vi "Insert UI into Subpanel.vi"(8 "error in":errorcluster, 11 "Philips Subpanel in":refnum<class "Flex UI Subpanel.lvclass">) -> (0 "error out":errorcluster, 3 "Philips Subpanel out":refnum<class "Flex UI Subpanel.lvclass">)   [LabVIEW 2014, in "Flex UI Subpanel.lvclass"]
uses:
  Flex UI Subpanel.lvclass
  Flex UI Subpanel.lvclass/Flex UI Subpanel.ctl
  Flex UI (Parent)/Flex UI.lvclass/Flex UI.ctl
  Flex UI (Parent)/Flex UI.lvclass
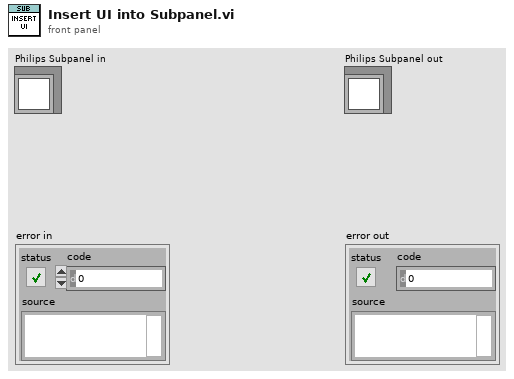
[diagram p1: front panel]
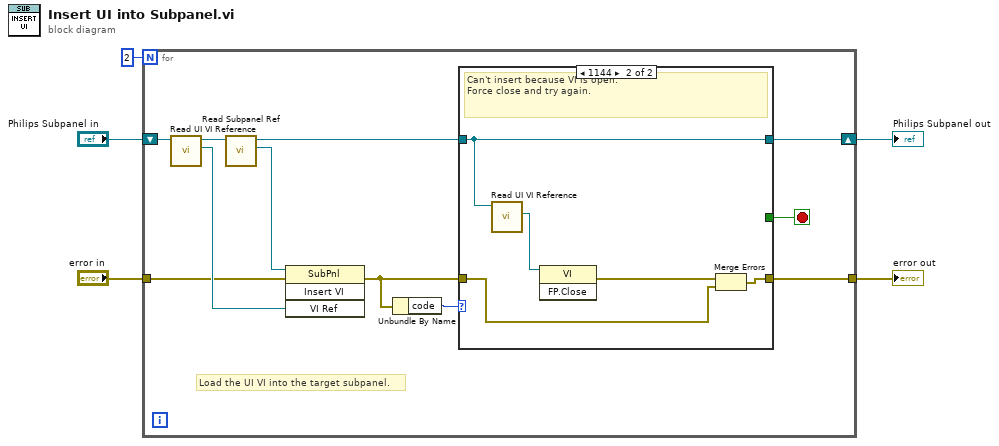
[diagram p0: block diagram]
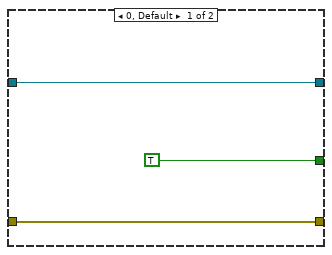
[diagram p2: hidden frame]
diagram:
  n1 = for {
    N: 2 -> [_]
    shift-right: [w9] -> w4
    shift-left: "Philips Subpanel in" -> [w16]
    tunnel: "error in" -> [w12]
    tunnel: [w7] -> w3
    stop <- w6 stop-if-true
    # "Load the UI VI into the target subpanel."
    n2 = call "Read UI VI Reference.vi"("Philips UI in"=w16) -> ("UI VI Reference"=w15:refnum<vi>, "Philips UI out"=w13:refnum<class "Flex UI Subpanel.lvclass">)  [unwired: 9 in]
    n3 = call "Read Subpanel Ref.vi"("Philips Subpanel in"=w13) -> ("Subpanel Ref"=w14:refnum<vi>, "Philips Subpanel out"=w10:refnum<class "Flex UI Subpanel.lvclass">)  [unwired: 9 in]
    n4 = invoke class="SubPnl" method="Insert VI"(reference=w14, error in=w12, "VI Ref"=w15) -> (error out=w8:errorcluster)  [unwired: 1 in, 3 out]
    n5 = Unbundle By Name(w8) -> ("code"=w11:i32)
    n6 = case shown="1144" w11 {
      tunnel: [w19 w24] -> w9
      tunnel: w10 -> [w19 w24]
      tunnel: [w18 w21] -> w7
      tunnel: w8 -> [w18 w20]
      tunnel: [TRUE _] -> w6
      frame 0, Default {
      }
      frame 1144 {
        # "Can't insert because VI is open.\nForce close and try again."
        n7 = call "Read UI VI Reference.vi"("Philips UI in"=w24) -> ("UI VI Reference"=w22:refnum<vi>)  [unwired: 9 in, 1 out]
        n8 = invoke class="VI" method="FP.Close"(reference=w22) -> (error out=w23:errorcluster)  [unwired: 2 in, 2 out]
        n9 = Merge Errors(w23, w20) -> (w21:errorcluster)
      }
    }
  }
  "Philips Subpanel out" <- w4
  "error out" <- w3
